vi "AlkInjPrimary.vi"() -> (0 "Alk Index2":u8[](array[numeric]), 1 "Alk Index1":u8[](array[numeric]), 2 "Alk Press2":u8[](array[numeric]), 3 "Alk Press1":u8[](array[numeric]), 4 "Dim1":i32, 5 "Dim2":i32, 6 "Alk Vent2":u8[](array[numeric]), 7 "Alk Vent1":u8[](array[numeric]), 8 "Alk Grow2":u8[](array[numeric]), 9 "Alk Grow1":u8[](array[numeric]))   [LabVIEW 2011]
uses:
  Globals/SysGlbs.vi
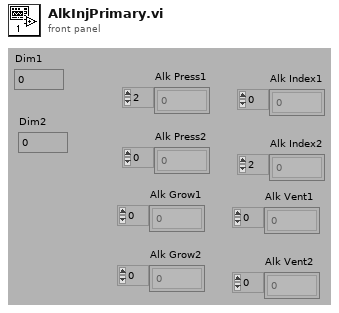
[diagram p1: front panel]
types:
  T1 = cluster{"Alk Index":u8[], "Alk Grow":u8[], "Alk Vent":u8[], "Alk Press":u8[], "Hyd Index":u8[], "Hyd Grow":u8[], "Hyd Vent":u8[], "Hyd Press":u8[], "Alk Primary":bool[], "Hyd Primary":bool[]}
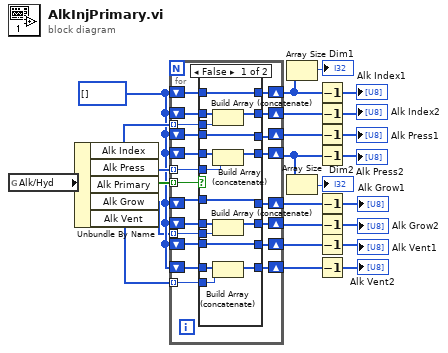
[diagram p0: block diagram]
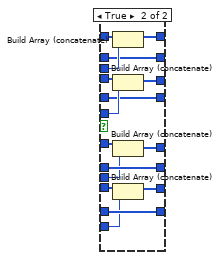
[diagram p2: hidden frame]
diagram:
  w11 = u8[] []
  n1 = global read "SysGlbs.vi" "Alk/Hyd"() -> (w25:T1)
  n2 = Unbundle By Name(w25) -> ("Alk Index"=w23:u8[], "Alk Press"=w22:u8[], "Alk Primary"=w24:bool[], "Alk Grow"=w9:u8[], "Alk Vent"=w10:u8[])
  n3 = for {
    shift-right: [w43] -> w19
    shift-left: w11 -> [w45]
    shift-right: [w41] -> w16
    shift-left: w11 -> [w42]
    shift-right: [w38] -> w17
    shift-left: w11 -> [w40]
    shift-right: [w36] -> w18
    shift-left: w11 -> [w37]
    tunnel: w24 -> [w46] mode=indexing
    tunnel: w23 -> [w44] mode=indexing
    tunnel: w22 -> [w39] mode=indexing
    shift-right: [w33] -> w8
    shift-left: w11 -> [w35]
    shift-right: [w30] -> w6
    shift-left: w11 -> [w31]
    shift-right: [w32] -> w7
    shift-left: w11 -> [w34]
    shift-right: [w28] -> w5
    shift-left: w11 -> [w29]
    tunnel: w10 -> [w27] mode=indexing
    tunnel: w9 -> [w26] mode=indexing
    n4 = case shown="False" w46 {
      tunnel: w45 -> [w62 w78]
      tunnel: w44 -> [w60 w77]
      tunnel: [w62 w76] -> w43
      tunnel: [w59 w75] -> w41
      tunnel: w42 -> [w61 w75]
      tunnel: w40 -> [w58 w74]
      tunnel: w39 -> [w56 w73]
      tunnel: [w58 w72] -> w38
      tunnel: [w55 w71] -> w36
      tunnel: w37 -> [w57 w71]
      tunnel: w35 -> [w54 w70]
      tunnel: w34 -> [w53 w69]
      tunnel: [w54 w68] -> w33
      tunnel: [w53 w67] -> w32
      tunnel: w31 -> [w52 w66]
      tunnel: [w50 w66] -> w30
      tunnel: w29 -> [w49 w65]
      tunnel: [w48 w65] -> w28
      tunnel: w27 -> [w47 w64]
      tunnel: w26 -> [w51 w63]
      frame False {
        n5 = Build Array (concatenate)(w61, w60) -> (w59:u8[])
        n6 = Build Array (concatenate)(w57, w56) -> (w55:u8[])
        n7 = Build Array (concatenate)(w52, w51) -> (w50:u8[])
        n8 = Build Array (concatenate)(w49, w47) -> (w48:u8[])
      }
      frame True {
        n9 = Build Array (concatenate)(w78, w77) -> (w76:u8[])
        n10 = Build Array (concatenate)(w74, w73) -> (w72:u8[])
        n11 = Build Array (concatenate)(w70, w63) -> (w68:u8[])
        n12 = Build Array (concatenate)(w69, w64) -> (w67:u8[])
      }
    }
  }
  n13 = Array Size(array=w19) -> (size(s)=→"Dim1":i32)
  n14 = Array Size(array=w18) -> (size(s)=→"Dim2":i32)
  n15 = Decrement(x=w19) -> (x-1=→"Alk Index1":u8[])
  n16 = Decrement(x=w16) -> (x-1=→"Alk Index2":u8[])
  n17 = Decrement(x=w17) -> (x-1=→"Alk Press1":u8[])
  n18 = Decrement(x=w18) -> (x-1=→"Alk Press2":u8[])
  n19 = Decrement(x=w8) -> (x-1=→"Alk Grow1":u8[])
  n20 = Decrement(x=w6) -> (x-1=→"Alk Grow2":u8[])
  n21 = Decrement(x=w7) -> (x-1=→"Alk Vent1":u8[])
  n22 = Decrement(x=w5) -> (x-1=→"Alk Vent2":u8[])
